vi "update.vi"(8 "deltaX":dbl, 9 "Alpha":dbl, 11 "X":dbl) -> (1 "X'":dbl)   [LabVIEW 2014]
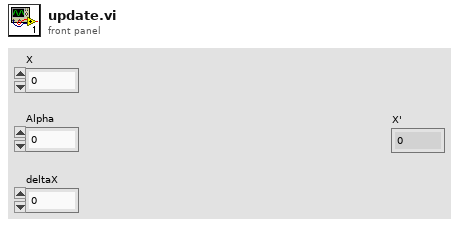
[diagram p1: front panel]
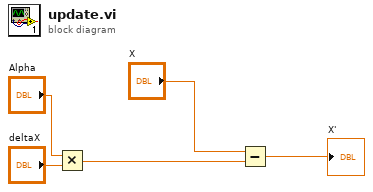
[diagram p0: block diagram]
diagram:
  n1 = Multiply(x="Alpha", y="deltaX") -> (x*y=w2:dbl)
  n2 = Subtract(x="X", y=w2) -> (x-y=→"X'":dbl)
